vi "CC Get Current Device.vi"(8 "error in (no error)":errorcluster, 10 "Device Type Name":string, 11 "Hardware.Installed Hardware":T1[](array[typedef])) -> (0 "error out":errorcluster, 2 "All Instances":string[](array[string]), 3 "Curr Device Name":string)   [LabVIEW 2021]
uses:
  typedefs/CC cluster Device Index.ctl
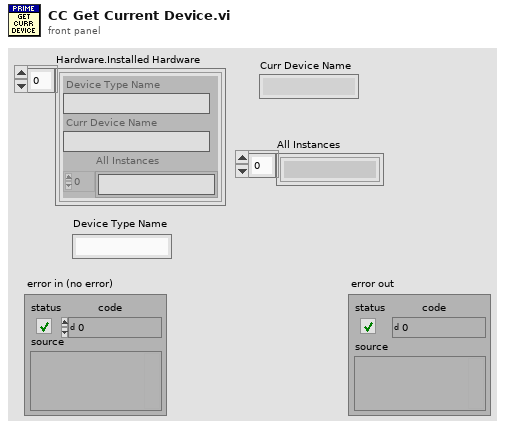
[diagram p1: front panel]
types:
  T1 = typedef "CC cluster Device Index.ctl" = cluster{"Device Type Name":string, "Curr Device Name":string, "All Instances":string[]}
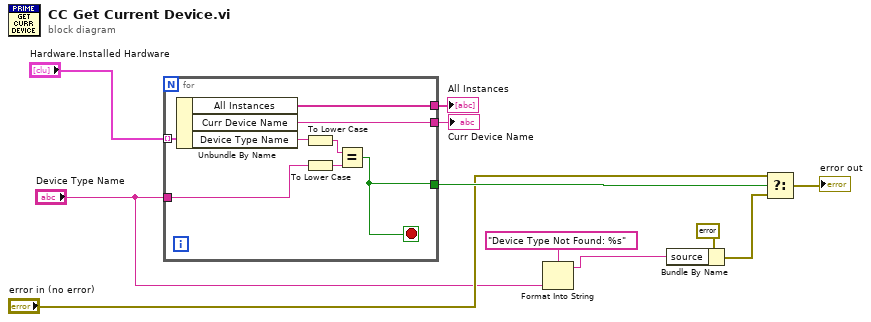
[diagram p0: block diagram]
diagram:
  n1 = for {
    tunnel: "Hardware.Installed Hardware" -> [w19] mode=indexing
    tunnel: "Device Type Name" -> [w17]
    tunnel: [w14] -> w9
    tunnel: [w13] -> w10
    tunnel: [w12] -> w8
    stop <- w12 stop-if-true
    n2 = Unbundle By Name(w19) -> ("All Instances"=w13:string[], "Curr Device Name"=w14:string, "Device Type Name"=w16:string)
    n3 = To Lower Case(string=w16) -> (all lower case string=w15:string)
    n4 = To Lower Case(string=w17) -> (all lower case string=w18:string)
    n5 = Equal?(x=w15, y=w18) -> (x = y?=w12:bool)
  }
  "All Instances" <- w10
  "Curr Device Name" <- w9
  n6 = Format Into String(format string="Device Type Not Found: %s", "Device Type Name") -> (resulting string=w4:string)  [unwired: 2 in, 1 out]
  n7 = Bundle By Name(cluster=errorcluster {"status"=TRUE, "code"=0, "source"=""} ("f"), "source"=w4) -> (w2:errorcluster)
  n8 = Select(t="error in (no error)", s=w8, f=w2) -> (s? t:f=→"error out":errorcluster)
